vi "CalculatePercentTicks.vi"(9 "Percent":dbl, 10 "Down Position":dbl, 11 "Start Position":dbl) -> (3 "Out Ticks":dbl)   [LabVIEW 2015]
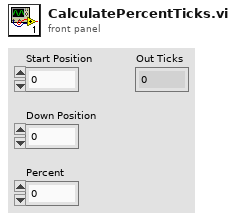
[diagram p1: front panel]
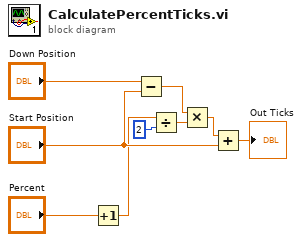
[diagram p0: block diagram]
diagram:
  n1 = Increment(x="Percent") -> (x+1=w3:dbl)
  n2 = Subtract(x="Down Position", y="Start Position") -> (x-y=w6:dbl)
  n3 = Divide(x=w3, y=2) -> (x/y=w2:dbl)
  n4 = Multiply(x=w6, y=w2) -> (x*y=w7:dbl)
  n5 = Add(x=w7, y="Start Position") -> (x+y=→"Out Ticks":dbl)
